vi "start.vi"(8 "error in (no error)":errorcluster, 11 "Model in":refnum<class "Model.lvclass">) -> (0 "error out":errorcluster, 3 "Model out":refnum<class "Model.lvclass">)   [LabVIEW 2013, in "Model.lvclass"]
uses:
  Model.lvclass
  Model.lvclass/Model.ctl
  <userlib>/Common/ILC/ILC/ILC.lvclass/ILC.ctl
  <userlib>/Common/ILC/ILC/ILC.lvclass
  <userlib>/Common/Devices/ForceSensorCalculator/ForceSensorCalculator/ForceSensorCalculator.lvclass
  ApplicationElements/SystemController/SystemController.lvclass
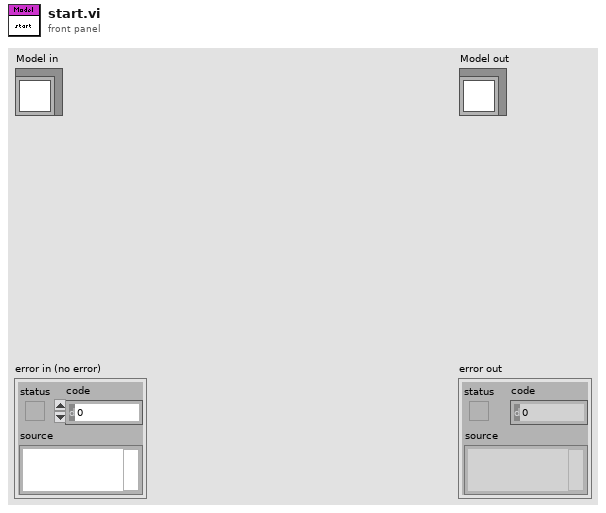
[diagram p1: front panel]
types:
  T1 = typedef "ILCCommon.lvlib/ILCConfiguration.lvlib/ILCADC.ctl" = cluster{"Input Channels":T2, "Scan Rate (Hz) ":T3, "PGA Gain Coefficient":u8, "Reference Voltage Vref":dbl[unit], "Nominal Input Range in Counts":u32, "Preamplifier Gain":u8, "Conversion Settling Cycles":u16}
  T2 = typedef "ILCCommon.lvlib/ILCConfiguration.lvlib/InputChannels.ctl" = enum16{"Channel 0", "3 Channels", "5 Channels"}
  T3 = typedef "ILCCommon.lvlib/ILCConfiguration.lvlib/ScanRate_Hz_MultichannelOptions.ctl" = enum16{"50", "60", "100", "120", "200", "240", "300", "400", "480", "600", "1200", "2400", "4800"}
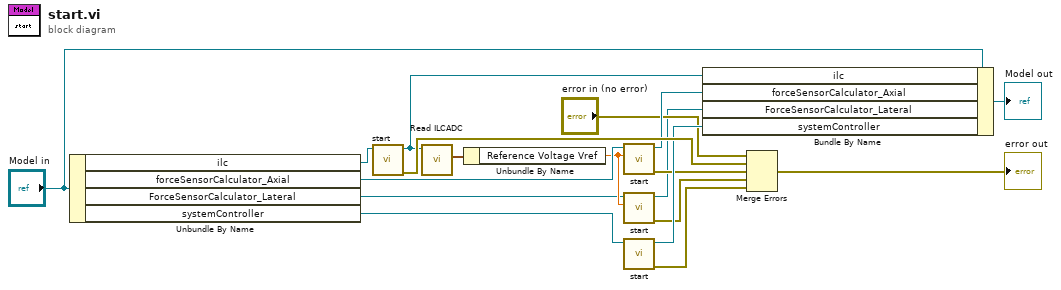
[diagram p0: block diagram]
diagram:
  n1 = Unbundle By Name("Model in") -> ("ilc"=w16:refnum<class "ILC.lvclass">, "forceSensorCalculator_Axial"=w13:refnum<class "ForceSensorCalculator_Axial.lvclass">, "ForceSensorCalculator_Lateral"=w2:refnum<class "ForceSensorCalculator_Lateral.lvclass">, "systemController"=w11:refnum<class "SystemController.lvclass">)
  n2 = call <userlib>:"start.vi"("ILC in"=w16) -> ("error out"=w15:errorcluster, "ILC out"=w5:refnum<class "ILC.lvclass">)  [unwired: 9 in]
  n3 = call <userlib>:"Read ILCADC.vi"("ILC in"=w5) -> ("ILC ADC"=w6:T1)  [unwired: 9 in, 1 out]
  n4 = Unbundle By Name(w6) -> ("Reference Voltage Vref"=w3:dbl[unit])
  n5 = call <userlib>:"start.vi"("Reference Voltage Vref"=w3, "ForceSensor in"=w13) -> ("error out"=w8:errorcluster, "ForceSensor out"=w12:refnum<class "ForceSensorCalculator_Axial.lvclass">)  [unwired: 8 in]
  n6 = call <userlib>:"start.vi"("Reference Voltage Vref"=w3, "ForceSensor in"=w2) -> ("error out"=w4:errorcluster, "ForceSensor out"=w1:refnum<class "ForceSensorCalculator_Lateral.lvclass">)  [unwired: 8 in]
  n7 = call <userlib>:"start.vi"("SystemController in"=w11) -> ("error out"=w7:errorcluster, "SystemController out"=w10:refnum<class "SystemController.lvclass">)  [unwired: 9 in]
  n8 = Bundle By Name(cluster="Model in", "ilc"=w5, "forceSensorCalculator_Axial"=w12, "ForceSensorCalculator_Lateral"=w1, "systemController"=w10) -> (→"Model out":refnum<class "Model.lvclass">)
  n9 = Merge Errors("error in (no error)", w15, w8, w4, w7) -> (→"error out":errorcluster)
